vi "KB numeric.vi"(10 "Parameters name":string) -> (1 "cancel?":bool, 2 "password":string)   [LabVIEW 2020]
panel:
  in  "Minus":bool
  in  "Exit":bool
  in  "dot":bool
  out "title":string
  in  "numbers":T1(radio)
  # "Enter Pass..."
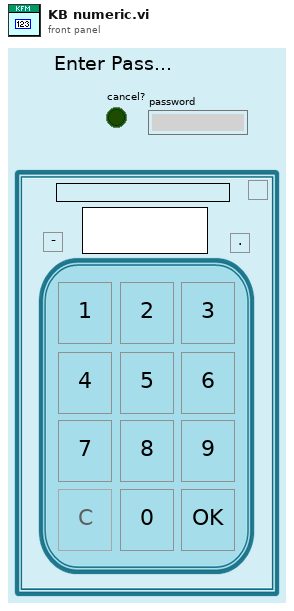
[diagram p1: front panel]
types:
  T1 = enum32{"No Selection", "1 10", "1", "1 2", "1 3", "1 4", "1 5", "1 6", "1 7", "1 8", "1 9", "1 11", "1 12"}
  T2 = enum8{"Enabled", "Disabled", "Disabled and Grayed Out"}
  T3 = enum32{"No Selection", "1", "1 2", "1 3", "1 4", "1 5", "1 6", "1 7", "1 8", "1 9", "1 10", "1 11", "1 12"}
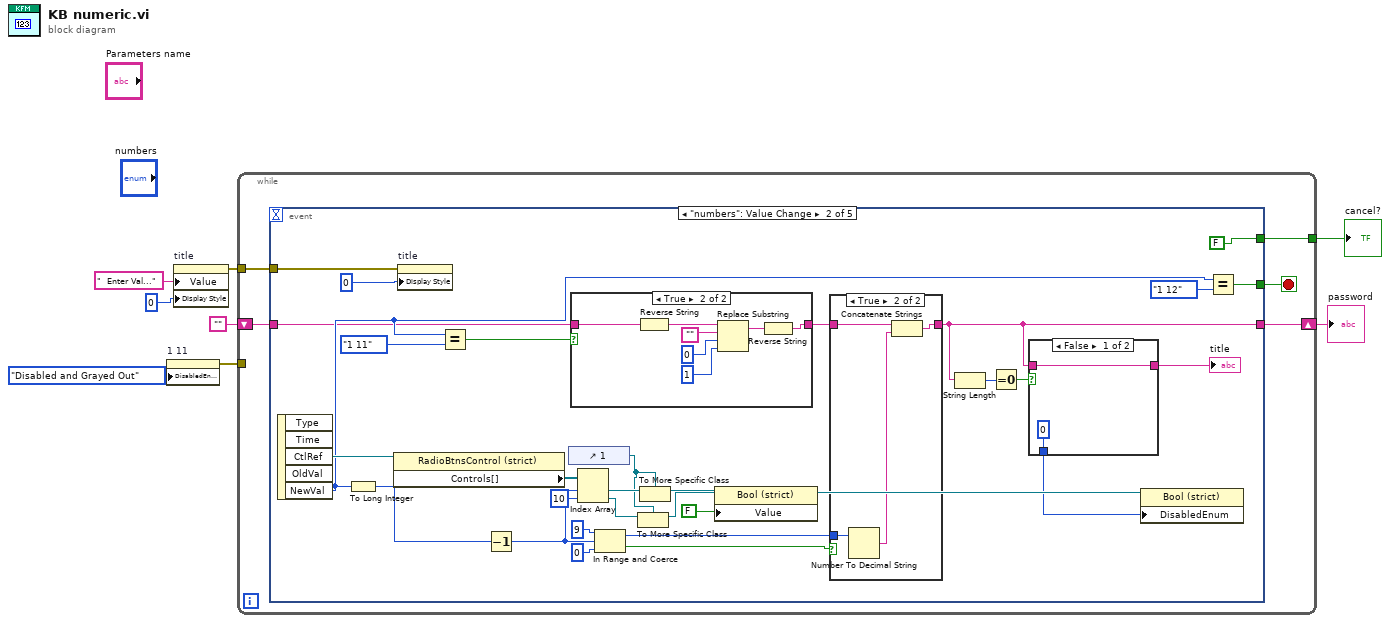
[diagram p0: block diagram]
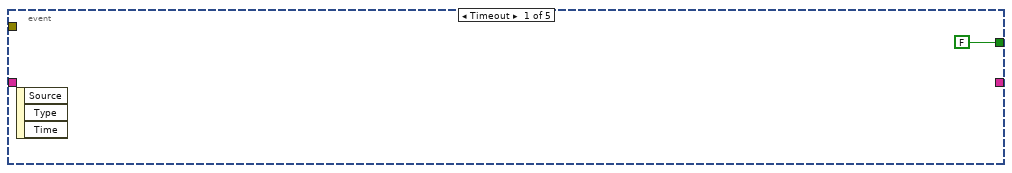
[diagram p2: hidden frame]
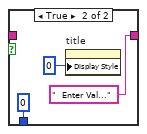
[diagram p3: hidden frame]
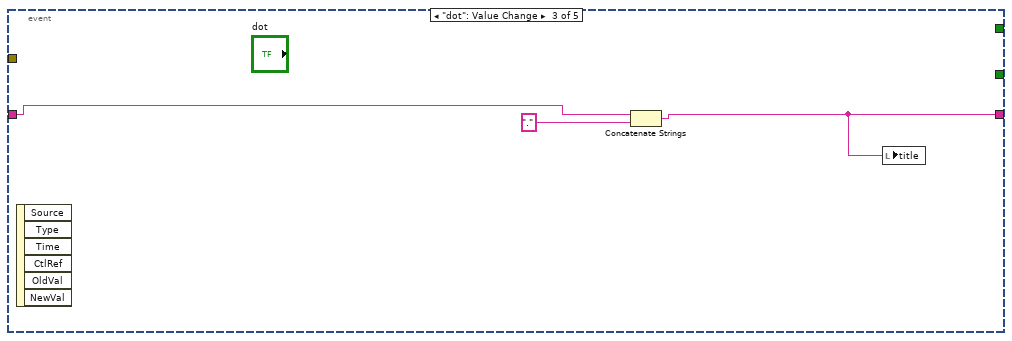
[diagram p6: hidden frame]
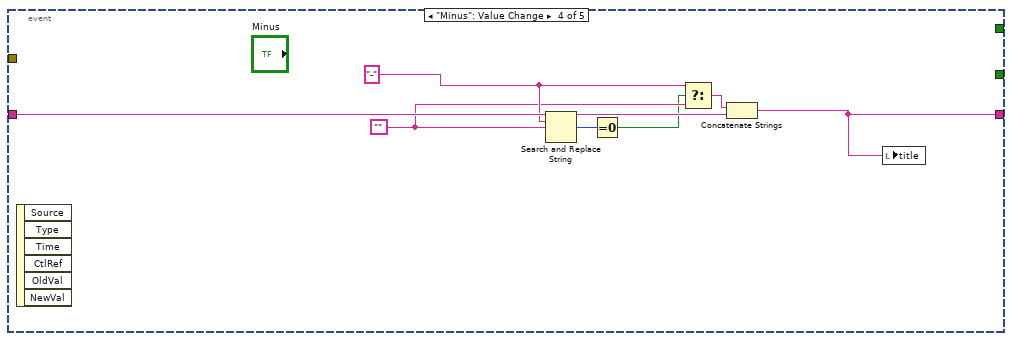
[diagram p7: hidden frame]
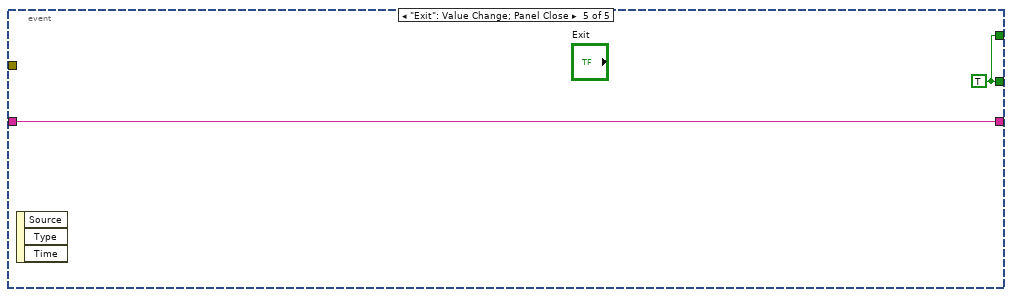
[diagram p8: hidden frame]
diagram:
  n1 = property on="1 11" class="Bool (strict)"("DisabledEnum"=T2."Disabled and Grayed Out" ("Disabled")) -> (error out=w2:errorcluster)  [unwired: 2 in, 1 out]
  n2 = property on="title" class="Str"("Value"="  Enter Val..." ("title"), "Display Style"=u32 0) -> (error out=w6:errorcluster)  [unwired: 2 in, 1 out]
  n3 = while {
    shift-right: [w11] -> w8
    shift-left: "" -> [w12]
    tunnel: w6 -> [w10]
    tunnel: w2 -> [_]
    tunnel: [w9] -> w1
    stop <- w13 stop-if-true
    n4 = event shown="[1] \"numbers\": Value Change" {
      selector: _ -> [_ _ _ _ _]
      dyn-events: _ -> [_ _ _ _ _]
      timeout: _ -> [_ _ _ _ _]
      tunnel: [FALSE w43 _ _ w75] -> w13
      tunnel: w12 -> [_ w30 w65 w72 w74]
      tunnel: [_ w22 w63 w73 w74] -> w11
      tunnel: w10 -> [_ w26 _ _ _]
      tunnel: [_ FALSE _ _ w75] -> w9
      event Timeout {
        n5 = event-data() -> ()  [unwired: 1 in, 3 out]
      }
      event "numbers": Value Change {
        n6 = event-data() -> ("CtlRef"=w42:refnum<vi>, "NewVal"=w32:T1)  [unwired: 1 in, 3 out]
        n7 = To Long Integer(number=w32) -> (32bit integer=w28:i32)
        n8 = property class="RadioBtnsControl (strict)"(reference=w42) -> ("Controls[]"=w41:refnum<vi>[])  [unwired: 1 in, 2 out]
        n9 = property on="title" class="Str"(error in=w26, "Display Style"=u32 0) -> ()  [unwired: 1 in, 2 out]
        n10 = Equal?(x=w32, y=T3."1 11") -> (x = y?=w31:bool)
        n11 = Decrement(x=w28) -> (x-1=w27:i32)
        n12 = control-ref of="1"() -> (w18:refnum<vi>)
        n13 = case shown="True" w31 {
          tunnel: w30 -> [w50 w57]
          tunnel: [w50 w51] -> w29
          frame False {
          }
          frame True {
            n14 = Reverse String(1:w57) -> (0:w56:string)
            n15 = Replace Substring(2:1 ("length (len. of substring)"), 3:0 ("offset (0)"), 4:"", 5:w56) -> (1:w52:string)  [unwired: 1 out]
            n16 = Reverse String(1:w52) -> (0:w51:string)
          }
        }
        n17 = Index Array(array=w41, index #1=w27, index #2=10 ("index")) -> (element #1=w40:refnum<vi>, element #2=w19:refnum<vi>)
        n18 = In Range and Coerce(upper limit=9, x=w27, lower limit=0) -> (coerced(x)=w34:i32, In Range?=w35:bool)
        n19 = To More Specific Class(target class=w18, reference=w19) -> (specific class reference=w17:refnum<vi>)  [unwired: 1 in, 1 out]
        n20 = To More Specific Class(target class=w18, reference=w40) -> (specific class reference=w38:refnum<vi>)  [unwired: 1 in, 1 out]
        n21 = property class="Bool (strict)"(reference=w38, "Value"=FALSE) -> ()  [unwired: 1 in, 2 out]
        n22 = case shown="True" w35 {
          tunnel: w34 -> [_ w62]
          tunnel: [w58 w61] -> w22
          tunnel: w29 -> [w58 w59]
          frame False {
          }
          frame True {
            n23 = Number To Decimal String(number=w62) -> (decimal integer string=w60:string)  [unwired: 1 in]
            n24 = Concatenate Strings(w59, w60) -> (w61:string)
          }
        }
        n25 = String Length(string=w22) -> (length=w24:i32)
        n26 = Equal To 0?(x=w24) -> (x = 0?=w23:bool)
        n27 = case shown="False" w23 {
          tunnel: w22 -> [w46 _]
          tunnel: [w46 "  Enter Val..." ("title")] -> w21
          tunnel: [u32 0 ("Display Style") u32 0 ("Display Style")] -> w16
          frame False {
          }
          frame True {
            n28 = property on="title" class="Str"("Display Style"=u32 0) -> ()  [unwired: 2 in, 2 out]
          }
        }
        "title" <- w21
        n29 = property class="Bool (strict)"(reference=w17, "DisabledEnum"=w16) -> ()  [unwired: 1 in, 2 out]
        n30 = Equal?(x=w32, y=T3."1 12") -> (x = y?=w43:bool)
      }
      event "dot": Value Change {
        n31 = event-data() -> ()  [unwired: 1 in, 6 out]
        n32 = Concatenate Strings(w65, "." ("title")) -> (w63:string)
        n33 = local write "title"(w63) -> ()
      }
      event "Minus": Value Change {
        w70 = ""
        w71 = "-" ("title")
        n34 = event-data() -> ()  [unwired: 1 in, 6 out]
        n35 = Search and Replace String(input string=w72, search string=w71, replace string=w70) -> (result string=w68:string, number of replacements=w67:i32)  [unwired: 5 in, 2 out]
        n36 = Equal To 0?(x=w67) -> (x = 0?=w66:bool)
        n37 = Select(t=w71, s=w66, f=w70) -> (s? t:f=w69:string)
        n38 = Concatenate Strings(w69, w68) -> (w73:string)
        n39 = local write "title"(w73) -> ()
      }
      event "Exit": Value Change; Panel Close {
        w75 = TRUE
        n40 = event-data() -> ()  [unwired: 1 in, 3 out]
      }
    }
  }
  "password" <- w8
  "cancel?" <- w1
